vi "Read Temp Module.vi"(7 "Temp Chan":string="T8", 8 "error in (no error)":errorcluster, 11 "Device":string(combo)="Elsa") -> (0 "error out":errorcluster, 3 "Temperature K":dbl)   [LabVIEW 2024]
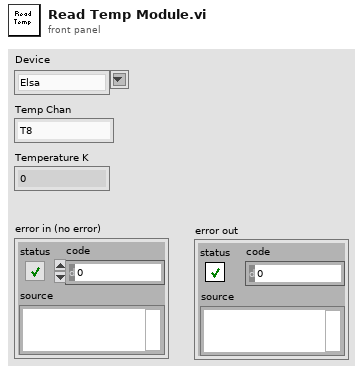
[diagram p1: front panel]
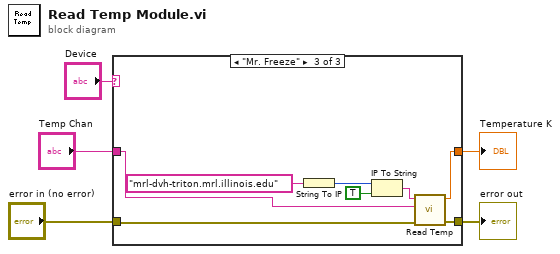
[diagram p0: block diagram]
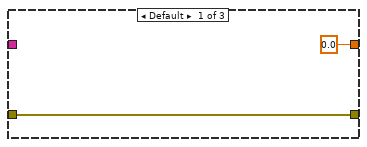
[diagram p2: hidden frame]
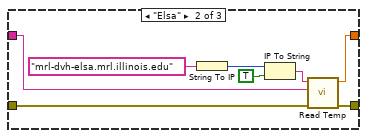
[diagram p3: hidden frame]
diagram:
  n1 = case shown="\"Mr. Freeze\"" "Device" {
    tunnel: "error in (no error)" -> [w6 w10 w17]
    tunnel: "Temp Chan" -> [_ w11 w16]
    tunnel: [w6 w9 w18] -> w2
    tunnel: [0.0 ("Temperature") w8 w19] -> w1
    frame Default {
    }
    frame "Elsa" {
      n2 = String To IP(1:"mrl-dvh-elsa.mrl.illinois.edu" ("name")) -> (0:w14:u32)
      n3 = IP To String(1:TRUE ("dot notation? (F)"), 2:w14) -> (0:w12:string)
      n4 = call "Read Temp.vi"("error in (no error)"=w10, "Temp Chan"=w11, "IP Address in"=w12) -> ("error out"=w9:errorcluster, "Temperature"=w8:dbl)  [unwired: 7 in]
    }
    frame "Mr. Freeze" {
      n5 = String To IP(1:"mrl-dvh-triton.mrl.illinois.edu" ("name")) -> (0:w22:u32)
      n6 = IP To String(1:TRUE ("dot notation? (F)"), 2:w22) -> (0:w23:string)
      n7 = call "Read Temp.vi"("error in (no error)"=w17, "Temp Chan"=w16, "IP Address in"=w23) -> ("error out"=w18:errorcluster, "Temperature"=w19:dbl)  [unwired: 7 in]
    }
  }
  "error out" <- w2
  "Temperature K" <- w1
